vi "mqttTCPIPbrokerConnect.vi"(0 "mqtt in":refnum<class "MQTT Client.lvclass">, 11 "error in (no error)":errorcluster) -> (4 "mqtt out":refnum<class "MQTT Client.lvclass">, 15 "error out":errorcluster)   [LabVIEW 2020, in "MQTT Client.lvclass"]
uses:
  MQTT Client.lvclass
  MQTT Client.lvclass/MQTT Client.ctl
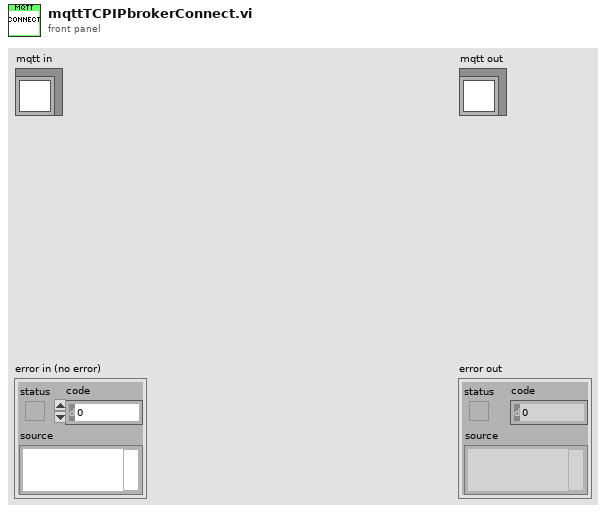
[diagram p1: front panel]
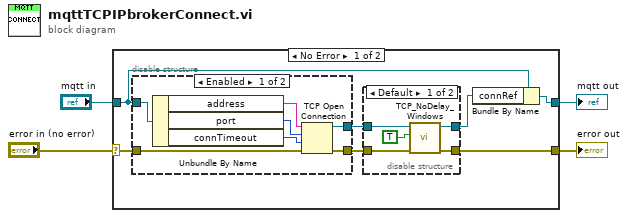
[diagram p0: block diagram]
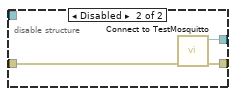
[diagram p2: hidden frame]
diagram:
  n1 = case shown="No Error" "error in (no error)" {
    selector: "error in (no error)" -> [w6 w30]
    tunnel: [w9 w30] -> w3
    tunnel: [w7 w29] -> w1
    tunnel: "mqtt in" -> [w5 w29]
    frame No Error {
      n2 = disable-structure shown="Enabled" {
        disable-tunnel: [w18 w19] -> w11
        disable-tunnel: [w17 w20] -> w10
        disable-tunnel: w6 -> [w16 w21]
        disable-tunnel: w5 -> [w15 _]
        frame Enabled {
          n3 = Unbundle By Name(w15) -> ("address"=w14:string, "port"=w13:u16, "connTimeout"=w12:i32)
          n4 = TCP Open Connection(address=w14, remote port or service name=w13, timeout ms (60000)=w12, error in (no error)=w16) -> (connection ID=w18:refnum<k5>, error out=w17:errorcluster)  [unwired: 1 in]
        }
        frame Disabled {
          n5 = call "Connect to TestMosquitto.vi"("error in"=w21) -> ("error out"=w20:errorcluster, "TCP Network Connection out"=w19:refnum<k5>)  [unwired: 8 in, 1 out]
        }
      }
      n6 = disable-structure shown="Default" {
        disable-tunnel: w11 -> [w26 w28]
        disable-tunnel: w10 -> [w25 w27]
        disable-tunnel: [w24 w27] -> w9
        disable-tunnel: [w22 w28] -> w8
        frame condition #0 (active) {
          n7 = call "TCP_NoDelay_Windows.vi"("error in (no error)"=w25, "TCP_NODELAY (true)"=TRUE, "connID"=w26) -> ("error out"=w24:errorcluster, "connID 2"=w22:refnum<k5>)  [unwired: 3 in]
        }
        frame condition #1 {
        }
      }
      n8 = Bundle By Name(cluster=w5, "connRef"=w8) -> (w7:refnum<class "MQTT Client.lvclass">)
    }
    frame Error {
    }
  }
  "error out" <- w3
  "mqtt out" <- w1
